vi "SubBus.vi"(6 "R":dbl, 9 "e3":bool, 10 "e2":bool, 11 "e1":bool) -> (2 "1-T/(R*e*C)":fxp<+,20,0>, 3 "T/(e*C)":fxp<+,20,0>)   [LabVIEW 2015]
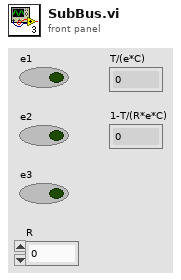
[diagram p1: front panel]
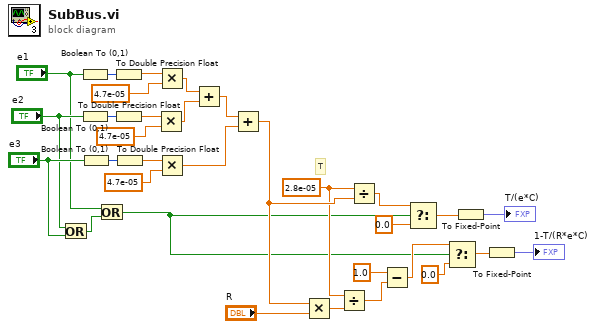
[diagram p0: block diagram]
diagram:
  w24 = 2.8e-05 ("x")
  # "T"
  n1 = Or(x="e2", y="e3") -> (x .or. y?=w5:bool)
  n2 = Boolean To (0,1)(Boolean="e1") -> (0, 1=w1:i16)
  n3 = Boolean To (0,1)(Boolean="e2") -> (0, 1=w2:i16)
  n4 = Boolean To (0,1)(Boolean="e3") -> (0, 1=w3:i16)
  n5 = Or(x="e1", y=w5) -> (x .or. y?=w8:bool)
  n6 = To Double Precision Float(number=w1) -> (double precision float=w10:dbl)
  n7 = To Double Precision Float(number=w2) -> (double precision float=w11:dbl)
  n8 = To Double Precision Float(number=w3) -> (double precision float=w12:dbl)
  n9 = Multiply(x=w11, y=4.7e-05) -> (x*y=w17:dbl)
  n10 = Multiply(x=w10, y=4.7e-05) -> (x*y=w16:dbl)
  n11 = Multiply(x=w12, y=4.7e-05) -> (x*y=w18:dbl)
  n12 = Add(x=w16, y=w17) -> (x+y=w9:dbl)
  n13 = Add(x=w9, y=w18) -> (x+y=w26:dbl)
  n14 = Multiply(x=w26, y="R") -> (x*y=w25:dbl)
  n15 = Divide(x=w24, y=w25) -> (x/y=w23:dbl)
  n16 = Divide(x=w24, y=w26) -> (x/y=w19:dbl)
  n17 = Subtract(x=1.0, y=w23) -> (x-y=w28:dbl)
  n18 = Select(t=w19, s=w8, f=0.0) -> (s? t:f=w21:dbl)
  n19 = Select(t=w28, s=w8, f=0.0) -> (s? t:f=w30:dbl)
  n20 = To Fixed-Point(number=w21) -> (fixed-point=→"T/(e*C)":fxp<+,20,0>)  [unwired: 1 in]
  n21 = To Fixed-Point(number=w30) -> (fixed-point=→"1-T/(R*e*C)":fxp<+,20,0>)  [unwired: 1 in]
